vi "Line Array to Cluster.vi"(11 "Array":string[](array[string])) -> (1 "Custom Roi":cluster{i32, i32, i32, i32, i32, i32}={0, 4096, 1, 0, 4096, 1}, 3 "cluster":T1={"SI camera info"={"Observer Name"="", "object name"="", "File name base"="", "Camera Color"="Red", "Exp type tab"=enum."Object", "Number of Exp"=1.0, "Exp time"=0.0, "CCD Readout Speed"=5, "CCD ROI Mode"=10, "Hg(Ar)"=FALSE, "Cu"=FALSE, "Ne"=FALSE, "Bulb"=FALSE, "Ar"=FALSE, "Quartz"=FALSE, "Quartz Percent"=0.0, "Fe"=FALSE, "Notes"="n", "Target Number"="", "Dome"=FALSE, "Dome Percent"=0.0}, "Configuration"={"Primary Filter"="<NO FILTER>", "Secondary Filter"="<NO FILTER>", "Slit Mask"="<NO MASK>", "Grating"="<NO GRATING>", "CS Target"=0.0, "GS Target"=0.0, "Coll Focus"=1000, "Camera Focus"=0, "Name"="", "User"="", "Date"="", "Comment"="", "use Flexure Comp?"=FALSE, "Select Mode:"=0}, "Path to Configuration File"=path ""} {"Configuration"."Select Mode:" items=["Custom", "Imaging", "300 All", "600 UV", "600 Blue", "600 Mid", "600 Red", "1200 m0", "1200 m1", "1200 m2", "1200 m3", "1200 m4", "1200 m5", "1200 m6", "1200 m7", "1200 RESOLVE", "400 m1", "400 m2", "930 m1", "930 m2", "930 m3", "930 m4", "930 m5", "930 m6", "400WD", "930TP", "400Fermi", "400Padgett", "400Lewis", "400Crotts", "600BLee", "600RLee", "400WW"]; "SI camera info"."Dome Percent" min=0.0 step=1.0; "SI camera info"."Quartz Percent" min=0.0 step=1.0; "SI camera info"."CCD Readout Speed" items=["750 kHz, ATTN 0", "750 kHz, ATTN 2", "344 kHz, ATTN 0", "344 kHz, ATTN 3", "100 kHz, ATTN 2", "100 kHz, ATTN 3"]; "SI camera info"."CCD ROI Mode" items=["Imaging, 1x1  "=0, "Imaging, 2x2"=1, "Imaging, 3x3"=2, "Spectroscopic, 1x1"=3, "Spectroscopic, 2x2"=4, "Spectroscopic, 3x3"=5, "MOS, 1x1"=11, "MOS, 2x2"=12, "MOS, 3x3"=13, "Slicer"=6, "Spectroscopic, ZZ Ceti"=14, "Slit Imaging/Alignment"=7, "MOS Imaging/Alignment"=10, "Set user-defined ROI..."=21, "Custom Mode"=9]; "SI camera info"."Number of Exp" min=1.0 step=1.0; "SI camera info"."Exp time" min=0.0 step=0.1})   [LabVIEW 2015]
panel:
  # "Or"
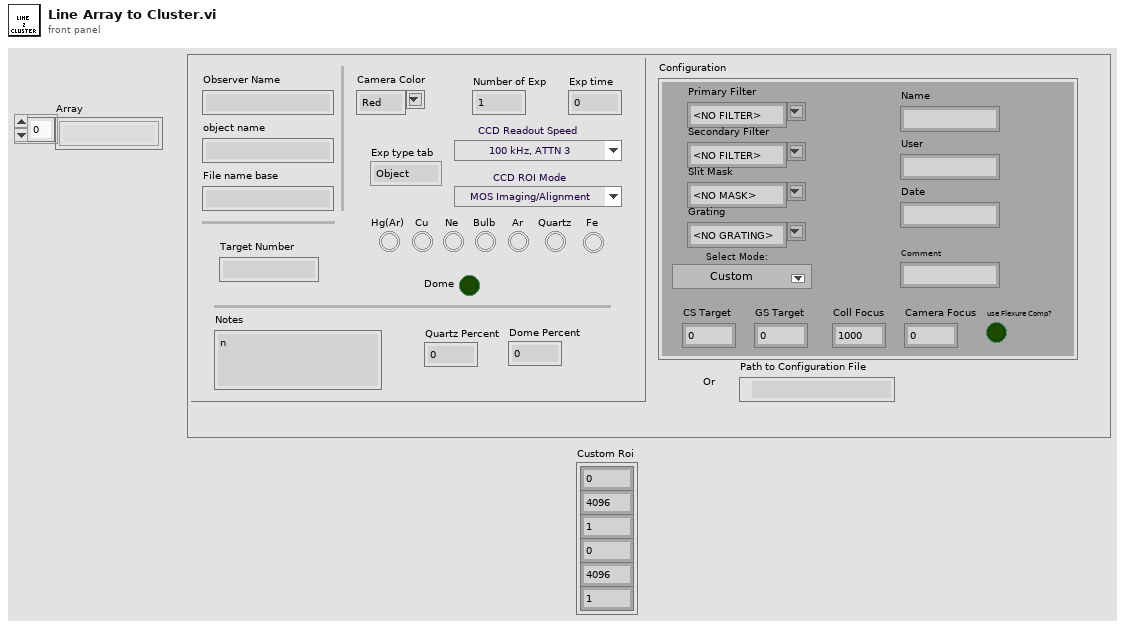
[diagram p1: front panel]
types:
  T1 = cluster{"SI camera info":cluster{"Observer Name":string, "object name":string, "File name base":string, "Camera Color":string, "Exp type tab":enum16{"Object", "Flat", "Comp", "Dark", "Zero"}, "Number of Exp":dbl, "Exp time":dbl, "CCD Readout Speed":u8, "CCD ROI Mode":u16, "Hg(Ar)":bool, "Cu":bool, "Ne":bool, "Bulb":bool, "Ar":bool, "Quartz":bool, "Quartz Percent":dbl, "Fe":bool, "Notes":string, "Target Number":string, "Dome":bool, "Dome Percent":dbl}, "Configuration":cluster{"Primary Filter":string, "Secondary Filter":string, "Slit Mask":string, "Grating":string, "CS Target":dbl, "GS Target":dbl, "Coll Focus":i32, "Camera Focus":i32, "Name":string, "User":string, "Date":string, "Comment":string, "use Flexure Comp?":bool, "Select Mode:":u16}, "Path to Configuration File":path}
  T2 = cluster{"[0]":string, "[1]":string, "[2]":string, "[3]":string, "[4]":string, "[5]":string, "[6]":string, "[7]":string, "[8]":string}
  T3 = cluster{"[0]":i32, "[1]":i32, "[2]":i32, "[3]":i32, "[4]":i32, "[5]":i32, "[6]":i32, "[7]":i32, "[8]":i32}
  T4 = cluster{"[0]":bool, "[1]":bool, "[2]":bool, "[3]":bool, "[4]":bool, "[5]":bool, "[6]":bool, "[7]":bool, "[8]":bool}
  T5 = typedef "configuration.ctl" = cluster{"Primary Filter":string, "Secondary Filter":string, "Slit Mask":string, "Grating":string, "CS Target":dbl, "GS Target":dbl, "Coll Focus":i32, "Camera Focus":i32, "Name":string, "User":string, "Date":string, "Comment":string, "use Flexure Comp?":bool, "Select Mode:":u16}
  T6 = cluster{"[0]":dbl, "[1]":dbl, "[2]":dbl, "[3]":dbl, "[4]":dbl, "[5]":dbl, "[6]":dbl, "[7]":dbl, "[8]":dbl}
  T7 = cluster{"[0]":i32, "[1]":i32, "[2]":i32, "[3]":i32, "[4]":i32, "[5]":i32}
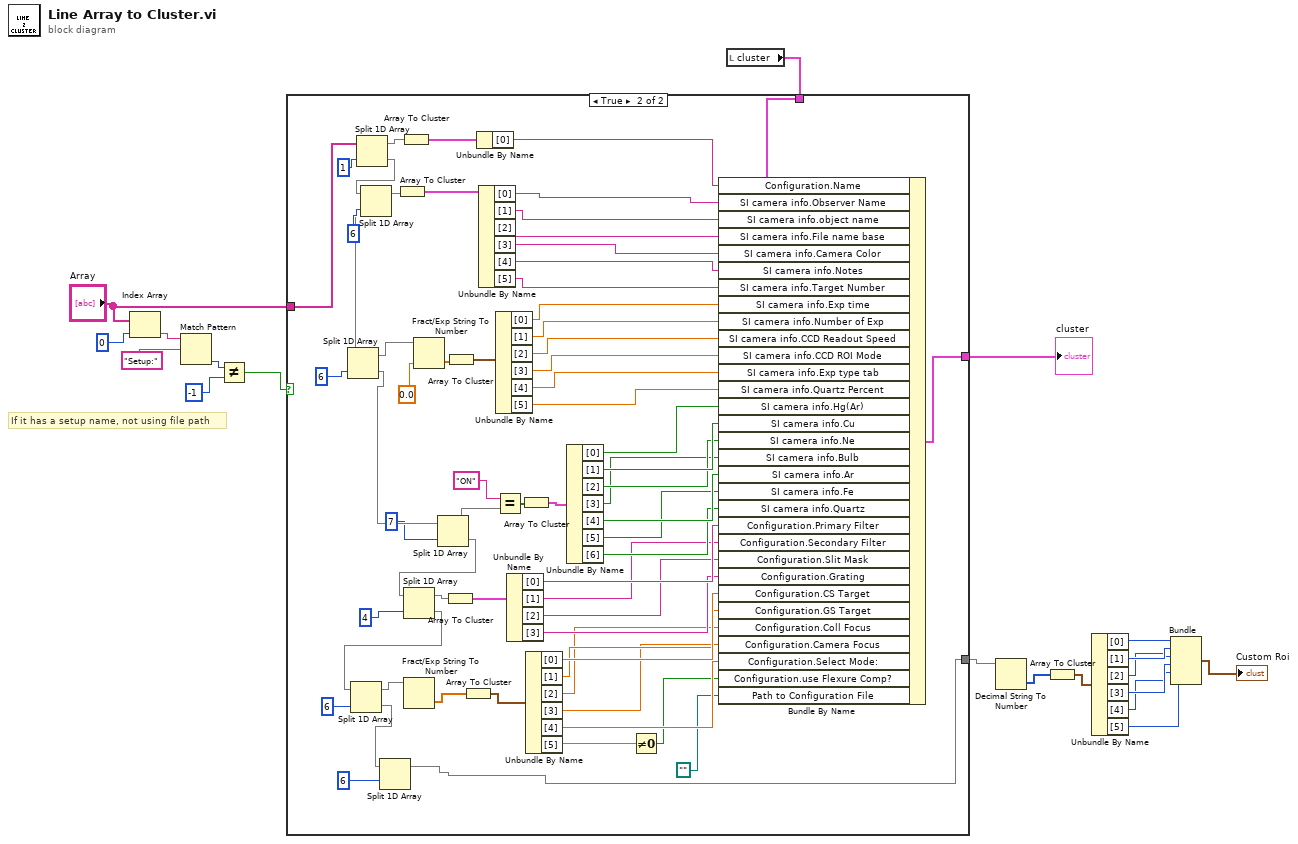
[diagram p0: block diagram]
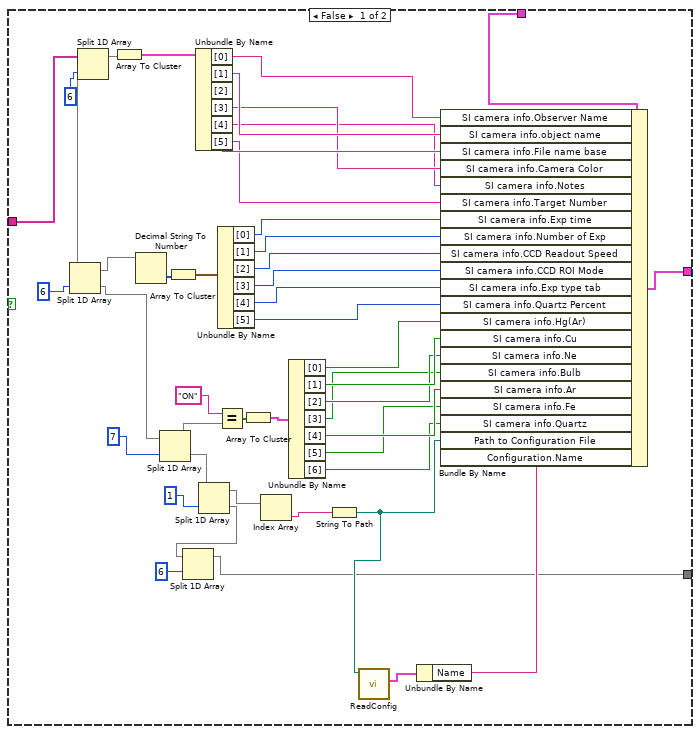
[diagram p2: hidden frame]
diagram:
  # "If it has a setup name, not using file path"
  n1 = Index Array(array="Array", index=0) -> (element=w18:string)
  n2 = Match Pattern(string=w18, regular expression="Setup:") -> (offset past match=w16:i32)  [unwired: 1 in, 3 out]
  n3 = Not Equal?(x=w16, y=-1) -> (x != y?=w14:bool)
  n4 = local read "cluster"() -> (w13:T1)
  n5 = case shown="True" w14 {
    tunnel: w13 -> [w65 w131]
    tunnel: "Array" -> [w64 w76]
    tunnel: [w30 w81] -> w11
    tunnel: [w21 w67] -> w9
    frame False {
      n6 = Split 1D Array(array=w64, index=6) -> (first subarray=w55:string[], second subarray=w62:string[])
      n7 = Split 1D Array(array=w62, index=6) -> (first subarray=w58:string[], second subarray=w60:string[])
      n8 = Array To Cluster(array=w55) -> (cluster=w54:T2)
      n9 = Decimal String To Number(string=w58) -> (number=w47:i32[])  [unwired: 2 in, 1 out]
      n10 = Split 1D Array(array=w60, index=7) -> (first subarray=w57:string[], second subarray=w26:string[])
      n11 = Array To Cluster(array=w47) -> (cluster=w46:T3)
      n12 = Unbundle By Name(w54) -> ("[0]"=w53:string, "[1]"=w52:string, "[2]"=w51:string, "[3]"=w50:string, "[4]"=w49:string, "[5]"=w48:string)
      n13 = Split 1D Array(array=w26, index=1) -> (first subarray=w25:string[], second subarray=w23:string[])
      n14 = Split 1D Array(array=w23, index=6) -> (first subarray=w21:string[])  [unwired: 1 out]
      n15 = Equal?(x="ON", y=w57) -> (x = y?=w39:bool[])
      n16 = Unbundle By Name(w46) -> ("[0]"=w45:i32, "[1]"=w44:i32, "[2]"=w43:i32, "[3]"=w42:i32, "[4]"=w41:i32, "[5]"=w40:i32)
      n17 = Array To Cluster(array=w39) -> (cluster=w38:T4)
      n18 = Index Array(array=w25) -> (element=w20:string)  [unwired: 1 in]
      n19 = Unbundle By Name(w38) -> ("[0]"=w37:bool, "[1]"=w36:bool, "[2]"=w35:bool, "[3]"=w34:bool, "[4]"=w33:bool, "[5]"=w32:bool, "[6]"=w31:bool)
      n20 = String To Path(string=w20) -> (path=w29:path)
      n21 = call "ReadConfig.vi"("configuration file path"=w29) -> ("Configuration"=w28:T5)  [unwired: 3 in, 3 out]
      n22 = Unbundle By Name(w28) -> ("Name"=w27:string)
      n23 = Bundle By Name(cluster=w65, "SI camera info.Observer Name"=w53, "SI camera info.object name"=w52, "SI camera info.File name base"=w51, "SI camera info.Camera Color"=w50, "SI camera info.Notes"=w49, "SI camera info.Target Number"=w48, "SI camera info.Exp time"=w45, "SI camera info.Number of Exp"=w44, "SI camera info.CCD Readout Speed"=w43, "SI camera info.CCD ROI Mode"=w42, "SI camera info.Exp type tab"=w41, "SI camera info.Quartz Percent"=w40, "SI camera info.Hg(Ar)"=w37, "SI camera info.Cu"=w36, "SI camera info.Ne"=w35, "SI camera info.Bulb"=w34, "SI camera info.Ar"=w33, "SI camera info.Fe"=w32, "SI camera info.Quartz"=w31, "Path to Configuration File"=w29, "Configuration.Name"=w27) -> (w30:T1)
    }
    frame True {
      n24 = Split 1D Array(array=w76, index=1) -> (first subarray=w73:string[], second subarray=w75:string[])
      n25 = Split 1D Array(array=w75, index=6) -> (first subarray=w122:string[], second subarray=w129:string[])
      n26 = Split 1D Array(array=w129, index=6) -> (first subarray=w125:string[], second subarray=w127:string[])
      n27 = Array To Cluster(array=w122) -> (cluster=w121:T2)
      n28 = Array To Cluster(array=w73) -> (cluster=w72:T2)
      n29 = Fract/Exp String To Number(string=w125, default (0 dbl)=0.0) -> (number=w114:dbl[])  [unwired: 2 in, 1 out]
      n30 = Split 1D Array(array=w127, index=7) -> (first subarray=w124:string[], second subarray=w97:string[])
      n31 = Split 1D Array(array=w97, index=4) -> (first subarray=w95:string[], second subarray=w79:string[])
      n32 = Split 1D Array(array=w79, index=6) -> (first subarray=w78:string[], second subarray=w69:string[])
      n33 = Split 1D Array(array=w69, index=6) -> (first subarray=w67:string[])  [unwired: 1 out]
      n34 = Fract/Exp String To Number(string=w78) -> (number=w89:dbl[])  [unwired: 3 in, 1 out]
      n35 = Array To Cluster(array=w95) -> (cluster=w94:T2)
      n36 = Array To Cluster(array=w114) -> (cluster=w113:T6)
      n37 = Array To Cluster(array=w89) -> (cluster=w88:T6)
      n38 = Unbundle By Name(w72) -> ("[0]"=w71:string)
      n39 = Unbundle By Name(w121) -> ("[0]"=w120:string, "[1]"=w119:string, "[2]"=w118:string, "[3]"=w117:string, "[4]"=w116:string, "[5]"=w115:string)
      n40 = Equal?(x="ON", y=w124) -> (x = y?=w106:bool[])
      n41 = Unbundle By Name(w113) -> ("[0]"=w112:dbl, "[1]"=w111:dbl, "[2]"=w110:dbl, "[3]"=w109:dbl, "[4]"=w108:dbl, "[5]"=w107:dbl)
      n42 = Unbundle By Name(w94) -> ("[0]"=w93:string, "[1]"=w92:string, "[2]"=w91:string, "[3]"=w90:string)
      n43 = Array To Cluster(array=w106) -> (cluster=w105:T4)
      n44 = Unbundle By Name(w88) -> ("[0]"=w87:dbl, "[1]"=w86:dbl, "[2]"=w70:dbl, "[3]"=w85:dbl, "[4]"=w84:dbl, "[5]"=w83:dbl)
      n45 = Unbundle By Name(w105) -> ("[0]"=w104:bool, "[1]"=w103:bool, "[2]"=w102:bool, "[3]"=w101:bool, "[4]"=w100:bool, "[5]"=w99:bool, "[6]"=w98:bool)
      n46 = Not Equal To 0?(x=w83) -> (x != 0?=w82:bool)
      n47 = Bundle By Name(cluster=w131, "Configuration.Name"=w71, "SI camera info.Observer Name"=w120, "SI camera info.object name"=w119, "SI camera info.File name base"=w118, "SI camera info.Camera Color"=w117, "SI camera info.Notes"=w116, "SI camera info.Target Number"=w115, "SI camera info.Exp time"=w112, "SI camera info.Number of Exp"=w111, "SI camera info.CCD Readout Speed"=w110, "SI camera info.CCD ROI Mode"=w109, "SI camera info.Exp type tab"=w108, "SI camera info.Quartz Percent"=w107, "SI camera info.Hg(Ar)"=w104, "SI camera info.Cu"=w103, "SI camera info.Ne"=w102, "SI camera info.Bulb"=w101, "SI camera info.Ar"=w100, "SI camera info.Fe"=w99, "SI camera info.Quartz"=w98, "Configuration.Primary Filter"=w93, "Configuration.Secondary Filter"=w92, "Configuration.Slit Mask"=w91, "Configuration.Grating"=w90, "Configuration.CS Target"=w87, "Configuration.GS Target"=w86, "Configuration.Coll Focus"=w70, "Configuration.Camera Focus"=w85, "Configuration.Select Mode:"=w84, "Configuration.use Flexure Comp?"=w82, "Path to Configuration File"=path "") -> (w81:T1)
    }
  }
  "cluster" <- w11
  n48 = Decimal String To Number(string=w9) -> (number=w10:i32[])  [unwired: 2 in, 1 out]
  n49 = Array To Cluster(array=w10) -> (cluster=w8:T3)
  n50 = Unbundle By Name(w8) -> ("[0]"=w7:i32, "[1]"=w6:i32, "[2]"=w5:i32, "[3]"=w4:i32, "[4]"=w3:i32, "[5]"=w2:i32)
  n51 = Bundle("[0]"=w7, "[1]"=w6, "[2]"=w5, "[3]"=w4, "[4]"=w3, "[5]"=w2) -> (→"Custom Roi":T7)  [unwired: 1 in]
